vi "TESTE save variables.vi"() -> ()   [LabVIEW 2026]
uses:
  <userlib>/LV-TOML/lib/LV-TOML.lvlib
  8ffc5d12-5297-497f-bdc5-4af82e1320d6.vi
  <userlib>/LV-TOML/lib/Write TOML File (LV).vi
panel:
  out "Value":T1
  out "Missing elements":string[](array[string])
  out "error out":errorcluster
  in  "Énum":enum16{""}(ring)
  in  "Error if missing element":bool caption="Error if missing element (F)"
  in  "variables":T1
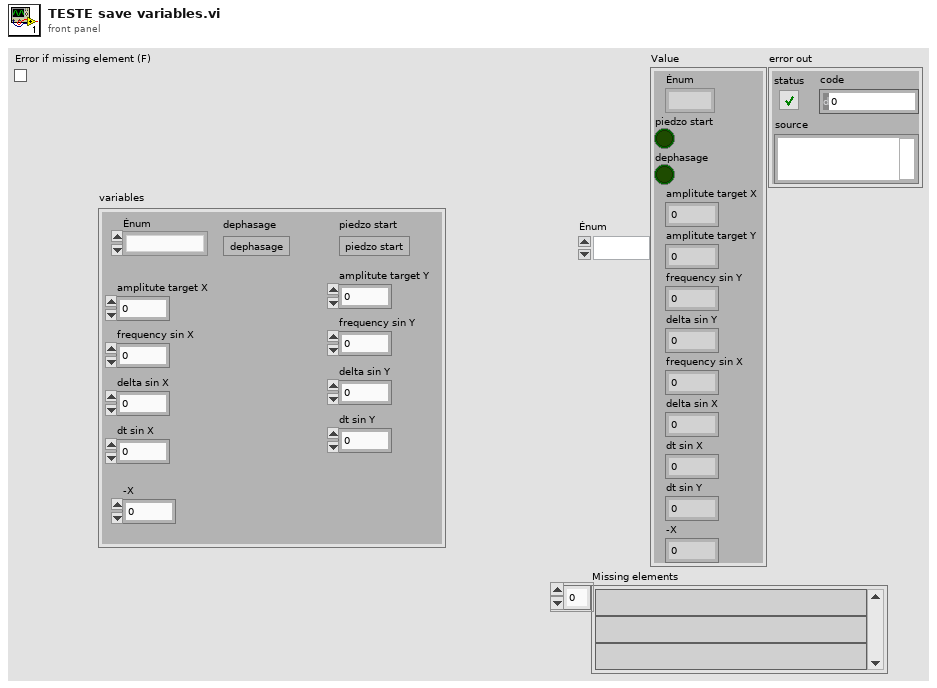
[diagram p1: front panel]
types:
  T1 = cluster{"Énum":enum16{""}, "piedzo start":bool, "dephasage":bool, "amplitute target X":dbl, "amplitute target Y":dbl, "frequency sin Y":dbl, "delta sin Y":dbl, "frequency sin X ":dbl, "delta sin X":dbl, "dt sin X":dbl, "dt sin Y":dbl, "-X":dbl}
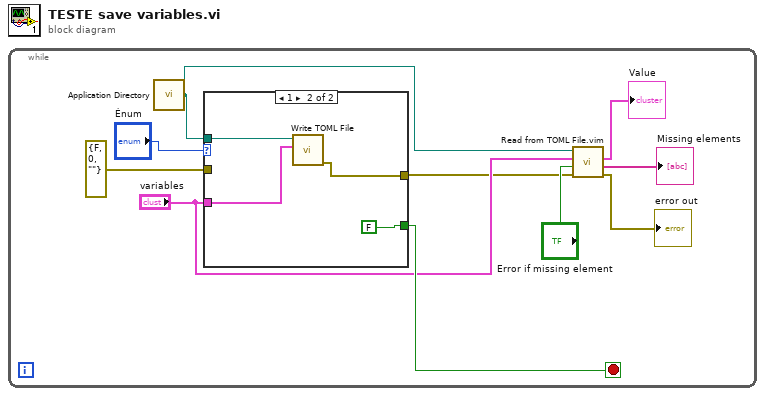
[diagram p0: block diagram]
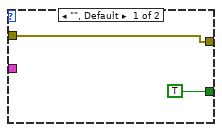
[diagram p2: hidden frame]
diagram:
  n1 = while {
    stop <- w8 stop-if-true
    n2 = call <vilib>:"Application Directory.vi"() -> ("Application Directory"=w7:path)
    n3 = case shown="\"1\"" "Énum" {
      tunnel: [TRUE FALSE] -> w8
      tunnel: w7 -> [_ w15]
      tunnel: "variables" -> [_ w14]
      tunnel: [w11 w13] -> w5
      tunnel: errorcluster {"status"=FALSE, "code"=0, "source"=""} ("error out") -> [w11 _]
      frame "", Default {
      }
      frame 1 {
        n4 = call-poly <userlib>:"Write TOML File.vi"("Value"=w14, "file path (use dialog)"=w15) -> ("error out"=w13:errorcluster)  [unwired: 9 in]
      }
    }
    n5 = call "Read from TOML File.vim"("error in (no error)"=w5, "Error if missing element"="Error if missing element", "Default Value"="variables", "file path (use dialog)"=w7) -> ("error out"=→"error out":errorcluster, "Missing elements"=→"Missing elements":string[], "Value"=→"Value":T1)  [unwired: 5 in]
  }
